vi "Append Report Text (str).vi"(0 "report in":refnum<class "NI_Word.lvclass">, 1 "MS Office parameters":T1, 2 "format string (%.3f)":string="%.3f", 7 "text":string, 9 "append on new line? (F)":bool, 11 "error in (no error)":errorcluster) -> (4 "report out":refnum<class "NI_Word.lvclass">, 8 "start out (Word)":i32, 10 "end out (Word)":i32, 15 "error out":errorcluster)   [LabVIEW 2020, in "NI_Word.lvclass"]
doc: "Appends text to the selected report."
uses:
  <vilib>/Utility/NIReport.llb/Word/NI_Word.lvclass
  <vilib>/Utility/NIReport.llb/Word/NI_Word.lvclass/NI_Word.ctl
  <vilib>/addons/_office/NI_ReportGenerationToolkit.lvlib
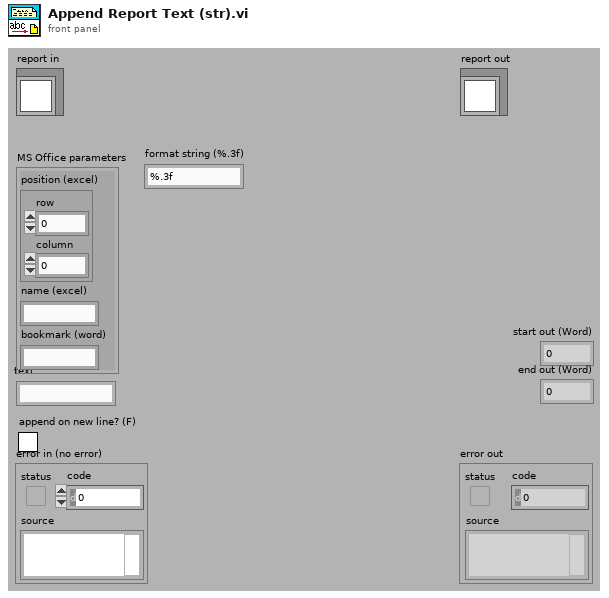
[diagram p1: front panel]
types:
  T1 = cluster{"position (excel)":cluster{"row":i32, "column":i32}, "name (excel)":string, "bookmark (word)":string}
  T2 = typedef "NI_ReportGenerationCore.lvlib/Report Data Members.ctl" = cluster{"font":T3, "from template?":bool}
  T3 = typedef "NI_ReportGenerationCore.lvlib/font.ctl" = cluster{"font name":string, "font size":dbl, "bold":u16, "italic":u16, "underline":u16, "strike through":u16, "font color":u32}
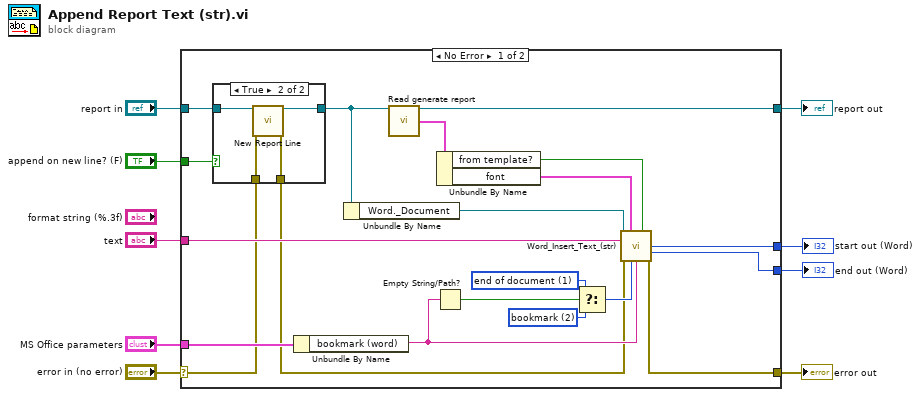
[diagram p0: block diagram]
diagram:
  n1 = case shown="No Error" "error in (no error)" {
    selector: "error in (no error)" -> [w16 w37]
    tunnel: [w19 w37] -> w8
    tunnel: [w13 w36] -> w6
    tunnel: "report in" -> [w29 w36]
    tunnel: "append on new line? (F)" -> [w28 _]
    tunnel: "MS Office parameters" -> [w21 _]
    tunnel: "text" -> [w20 _]
    tunnel: [w18 _] -> w2
    tunnel: [w17 _] -> w1
    frame No Error {
      w22 = u16 2 items=["begining of document", "end of document", "bookmark", "custom"] ("Insertion point")
      w23 = u16 1 items=["begining of document", "end of document", "bookmark", "custom"] ("Insertion point")
      n2 = case shown="True" w28 {
        tunnel: w29 -> [w31 w35]
        tunnel: [w31 w34] -> w14
        tunnel: w16 -> [w30 w33]
        tunnel: [w30 w32] -> w15
        frame False {
        }
        frame True {
          n3 = call-dynamic "New Report Line.vi"("report in"=w35, "error in (no error)"=w33) -> ("report out"=w34:refnum<class "NI_Word.lvclass">, "error out"=w32:errorcluster)  [unwired: 12 in]
        }
      }
      n4 = Unbundle By Name(w21) -> ("bookmark (word)"=w26:string)
      n5 = Unbundle By Name(w14) -> ("Word._Document"=w27:refnum<k7>)
      n6 = call-dynamic "Read generate report.vi"("report in"=w14) -> ("report out"=w13:refnum<class "NI_Word.lvclass">, "generate report"=w12:T2)  [unwired: 12 in, 1 out]
      n7 = Empty String/Path?(string/path=w26) -> (empty?=w24:bool)
      n8 = Unbundle By Name(w12) -> ("from template?"=w11:bool, "font"=w10:T3)
      n9 = Select(t=w23, s=w24, f=w22) -> (s? t:f=w25:u16)
      n10 = call <vilib>:"Word_Insert_Text_(str).vi"("Word._Document"=w27, "font"=w10, "from template?"=w11, "Text"=w20, "Error in (no error)"=w15, "Insertion point"=w25, "Bookmark name"=w26) -> ("Start out"=w18:i32, "End out"=w17:i32, "Error out"=w19:errorcluster)  [unwired: 3 in, 3 out]
    }
    frame Error {
    }
  }
  "error out" <- w8
  "report out" <- w6
  "start out (Word)" <- w2
  "end out (Word)" <- w1
